vi "ConfigureVariable.vi"(6 "Apply New Setpoint":bool, 8 "New Setpoint Value":dbl, 10 "Setpoint Save Location":path) -> (0 "Selected Setpoint Value":dbl)   [LabVIEW 2020]
uses:
  <vilib>/Utility/xml.llb/Write to XML File(string).vi
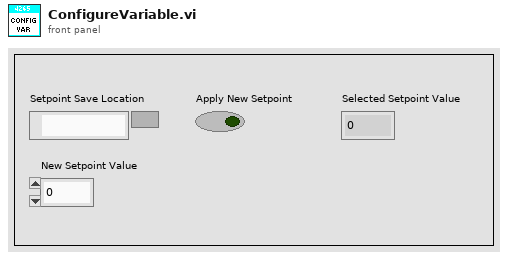
[diagram p1: front panel]
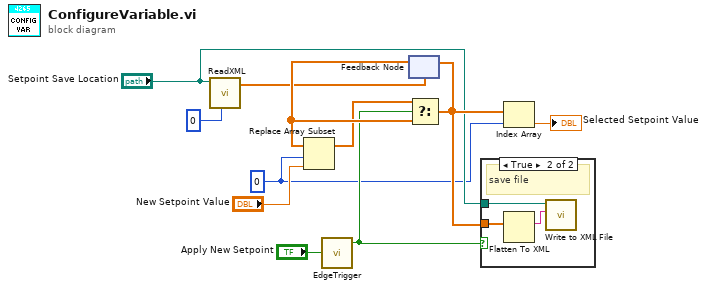
[diagram p0: block diagram]
diagram:
  w2 = 0 ("Selected Setpoint Index")
  n1 = call "ReadXML.vi"("Default Number of Elements"=0, "File Path (.xml)"="Setpoint Save Location") -> ("Data"=w3:dbl[])  [unwired: 8 in, 1 out]
  n2 = call "EdgeTrigger.vi"("Input Signal"="Apply New Setpoint") -> ("Rising Edge Trigger"=w7:bool)  [unwired: 2 out]
  n3 = feedback #1(w3) -> (w11:dbl[])
  n4 = Replace Array Subset(array=w11, new element="New Setpoint Value", index=w2) -> (w4:dbl[])
  n5 = Select(t=w4, s=w7, f=w11) -> (s? t:f=w9:dbl[])
  n6 = feedback-in #1(w9) -> ()
  n7 = case shown="True" w7 {
    tunnel: w9 -> [_ w13]
    tunnel: "Setpoint Save Location" -> [_ w12]
    frame False {
    }
    frame True {
      # "save file"
      n8 = Flatten To XML(6:w13) -> (2:w14:string)
      n9 = call-poly <vilib>:"Write to XML File.vi"("XML Input"=w14, "XML File Path"=w12) -> ()  [unwired: 7 in, 3 out]
    }
  }
  n10 = Index Array(array=w9, index=w2) -> (element=→"Selected Setpoint Value":dbl)
